vi "Begin.vi"(8 "error in":errorcluster) -> (0 "error out":errorcluster)   [LabVIEW 2017]
doc: "Called before other user functions, this VI is expected to open initial I/O refnums, load in file data, and do all program initialization. Notice that the <B>error out</B> terminal is simply used for data flow. Wiring it to other structures or subVIs ensures that this VI runs first."
uses:
  <vilib>/Rock Robotics/WPI/DriverStation/WPI_DriverStationRobotMode2.ctl
  <vilib>/Rock Robotics/WPI/Joystick/WPI_JoystickDeviceEnum.ctl
  <vilib>/Rock Robotics/WPI/Solenoid/WPI_SolenoidChannel.ctl
  <vilib>/Rock Robotics/WPI/SafetyOutput/WPI_SafetyOutputConfigMenu.ctl
  <vilib>/Rock Robotics/SystemInterfaces/DIO/FPGA_DIOPWMChannel.ctl
  Robot Global Data.vi
  <vilib>/Rock Robotics/Network Tables/NT Write String Array.vi
  <vilib>/Rock Robotics/WPI/MotorControl/WPI_MotorControlOpen VictorSP.vi
  <vilib>/Rock Robotics/WPI/Solenoid/WPI_SolenoidOpenDouble.vi
  <vilib>/Rock Robotics/WPI/RobotDrive/WPI_RobotDriveOpen2MotorWithExistingMotors.vi
  <vilib>/Rock Robotics/WPI/Utilities/WPI_GetSetVariantRefNum.vi
  <vilib>/Rock Robotics/WPI/MotorControl/WPI_MotorControlOpen SPARK.vi
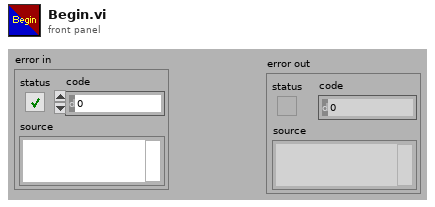
[diagram p1: front panel]
types:
  T1 = typedef "FPGA_DIOPWMChannel.ctl" = enum8{"PWM 0", "PWM 1", "PWM 2", "PWM 3", "PWM 4", "PWM 5", "PWM 6", "PWM 7", "PWM 8", "PWM 9", "PWM MXP 0", "PWM MXP 1", "PWM MXP 2", "PWM MXP 3", "PWM MXP 4", "PWM MXP 5", "PWM MXP 6", "PWM MXP 7", "PWM MXP 8", "PWM MXP 9", "Invalid"}
  T2 = typedef "WPI_SafetyOutputConfigMenu.ctl" = enum16{"Enable", "Disable"}
  T3 = typedef "WPI_SolenoidChannel.ctl" = enum8{"Solenoid 0", "Solenoid 1", "Solenoid 2", "Solenoid 3", "Solenoid 4", "Solenoid 5", "Solenoid 6", "Solenoid 7", "Invalid"}
  T4 = typedef "WPI_JoystickDeviceEnum.ctl" = enum16{"USB 0", "USB 1", "USB 2", "USB 3", "USB 4", "USB 5"}
  T5 = typedef "WPI_DriverStationRobotMode2.ctl" = enum16{"Autonomous Disabled", "Autonomous Enabled", "Teleop Disabled", "Teleop Enabled", "Disconnected", "Finish", "Test Disabled", "Test Enabled", "Emergency Stopped"}
  T6 = typedef "WPI_MotorControlDeviceRef.ctl" = cluster{"DeviceStatus":errorcluster, "Type":T7, "PWM":cluster{"PWM Channel":T1, "DeadBand":T8}, "CAN":cluster{"Device Number":u8, "SetOutput VI Ref":variant, "GetOutput VI Ref":variant, "Enable VI Ref":variant, "Disable VI Ref":variant, "Data":variant}, "Invert":bool, "DIO PWM":cluster{"PWM \"Enable\" Channel":T1, "DIOChannel":T9, "PWM Rate":dbl}}
  T7 = typedef "WPI_MotorControlType.ctl" = enum16{"PWM", "CAN", "DIO PWM"}
  T8 = typedef "WPI_PWMDeadband.ctl" = cluster{"Name":string, "maxPositivePwm":i32, "minPositivePwm":i32, "centerPwm":i32, "maxNegativePwm":i32, "minNegativePwm":i32, "angularRange":u16}
  T9 = typedef "FPGA_DIOChannel.ctl" = enum8{"DIO 0", "DIO 1", "DIO 2", "DIO 3", "DIO 4", "DIO 5", "DIO 6", "DIO 7", "DIO 8", "DIO 9", "DIO MXP 0", "DIO MXP 1", "DIO MXP 2", "DIO MXP 3", "DIO MXP 4", "DIO MXP 5", "DIO MXP 6", "DIO MXP 7", "DIO MXP 8", "DIO MXP 9", "DIO MXP 10", "DIO MXP 11", "DIO MXP 12", "DIO MXP 13", "DIO MXP 14", "DIO MXP 15", "SPI Port CS1", "SPI Port CS2", "SPI Port CS3", "SPI Port MISO", "SPI Port MOSI", "Invalid"}
  T10 = typedef "WPI_SolenoidDevRef.ctl" = cluster{"DevStatus":errorcluster, "Pneumatics Control Module":u8, "Forward Solenoid Channel":T3, "Reverse Solenoid Channel":T3}
  T11 = typedef "WPI_JoystickDevRef.ctl" = cluster{"Device":T4}
  T12 = typedef "WPI_RobotDriveDevRef.ctl" = cluster{"DevStatus":errorcluster, "Motors[]":T6[], "Square Inputs":bool, "Max Output":dbl}
  T13 = typedef "WPI_CompressorDevRef.ctl" = cluster{"DevStatus":errorcluster, "Pneumatics Control Module":u8}
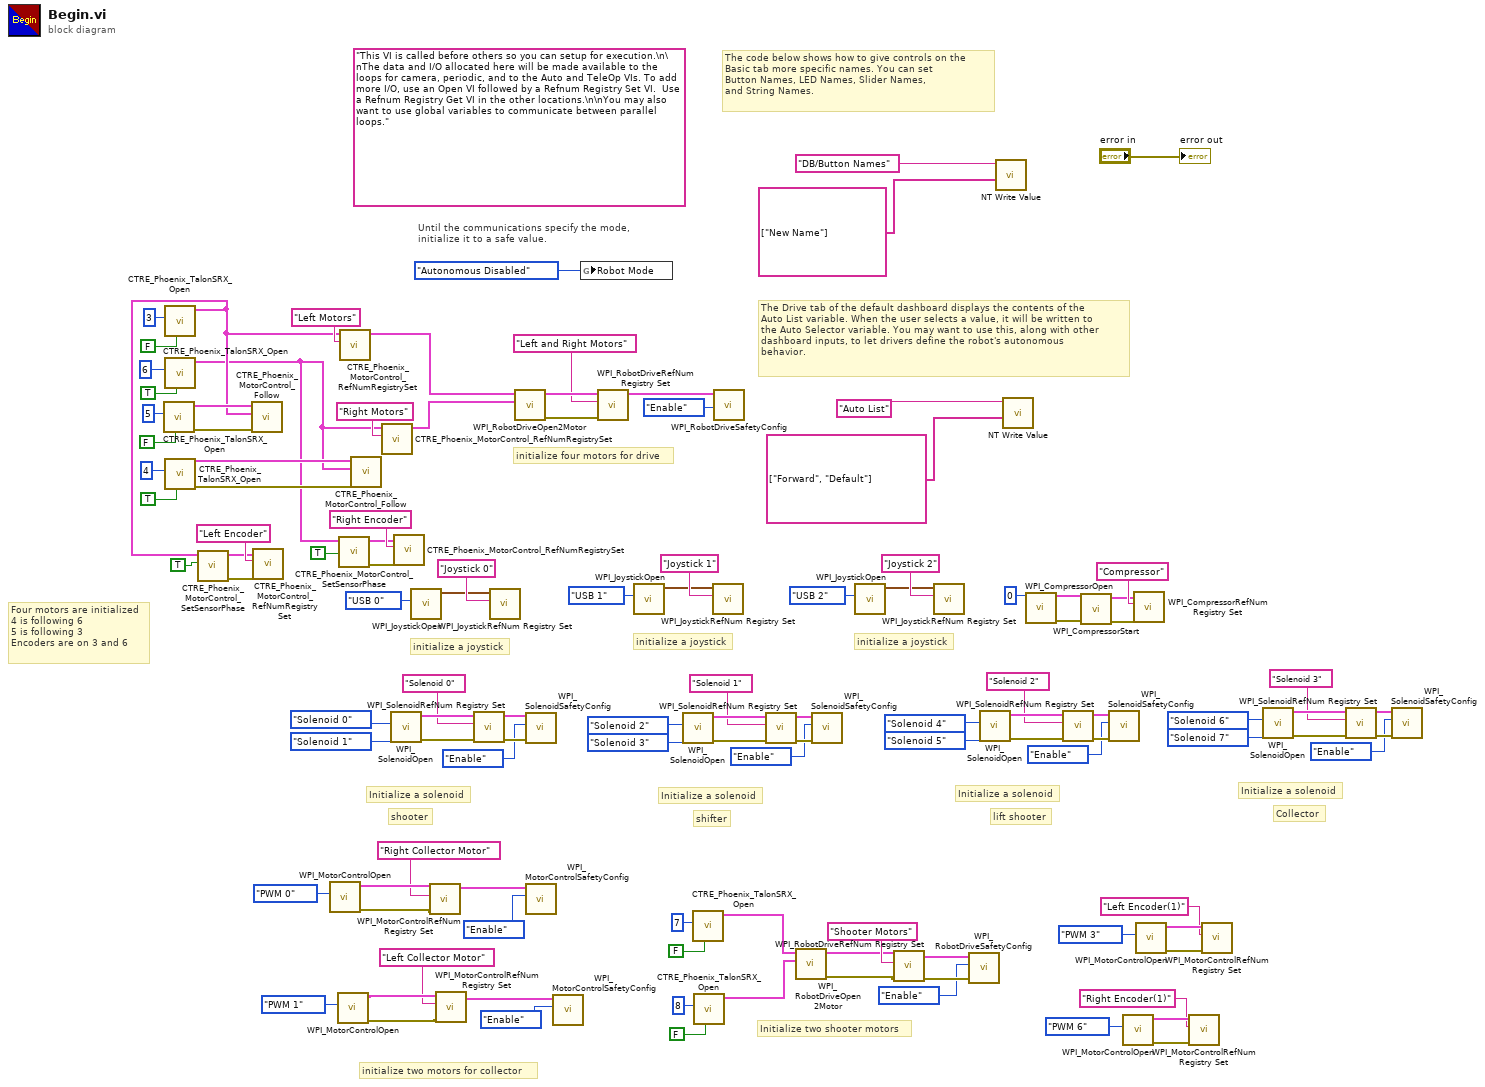
[diagram p0: block diagram]
diagram:
  (unwired) "This VI is called before others so you can setup for execution.\n\nThe data and I/O allocated here will be made available to the loops for camera, periodic, and to the Auto and TeleOp VIs. To add more I/O, use an Open VI followed by a Refnum Registry Set VI.  Use a Refnum Registry Get VI in the other locations.\n\nYou may also want to use global variables to communicate between parallel loops."
  # "Four motors are initialized\n4 is following 6\n5 is following 3\nEncoders are on 3 and 6"
  # "Initialize two shooter motors"
  # "Collector"
  # "Initialize a solenoid"
  # "lift shooter"
  # "Initialize a solenoid"
  # "initialize two motors for collector"
  # "shifter"
  # "shooter"
  # "Initialize a solenoid"
  # "Initialize a solenoid"
  # "initialize a joystick"
  # "initialize a joystick"
  # "The Drive tab of the default dashboard displays the contents of the\nAuto List variable. When the user selects a value, it will be written to\nthe Auto Selector variable. You may want to use this, along with other\ndashboard inputs, to let drivers define the robot's autonomous\nbehavior."
  # "The code below shows how to give controls on the\nBasic tab more specific names. You can set\nButton Names, LED Names, Slider Names,\nand String Names."
  # "initialize a joystick"
  # "Until the communications specify the mode,\ninitialize it to a safe value."
  # "initialize four motors for drive"
  n1 = call <vilib>:"CTRE_Phoenix_TalonSRX_Open.vi"("Invert"=FALSE, "Device Number"=u8 5) -> ("error out"=w56:errorcluster, "CAN Talon SRX Ref"=w55:T6)  [unwired: 8 in]
  n2 = call <vilib>:"CTRE_Phoenix_TalonSRX_Open.vi"("Invert"=FALSE, "Device Number"=u8 3) -> ("CAN Talon SRX Ref"=w43:T6)  [unwired: 8 in, 1 out]
  n3 = call <vilib>:"CTRE_Phoenix_TalonSRX_Open.vi"("Invert"=TRUE, "Device Number"=u8 6) -> ("CAN Talon SRX Ref"=w39:T6)  [unwired: 8 in, 1 out]
  n4 = call <vilib>:"CTRE_Phoenix_TalonSRX_Open.vi"("Invert"=TRUE, "Device Number"=u8 4) -> ("error out"=w53:errorcluster, "CAN Talon SRX Ref"=w54:T6)  [unwired: 8 in]
  n5 = call <vilib>:"CTRE_Phoenix_MotorControl_SetSensorPhase.vi"("PhaseSensor"=TRUE ("Invert"), "PhoenixMotorControlDevRef"=w43) -> ("error out"=w44:errorcluster, "PhoenixMotorControlDevRef"=w45:T6)  [unwired: 8 in]
  n6 = call <vilib>:"CTRE_Phoenix_MotorControl_Follow.vi"("error in (no error)"=w56, "Master Controller to Follow"=w43, "PhoenixMotorControlDevRef"=w55) -> ()  [unwired: 7 in, 2 out]
  n7 = call "CTRE_Phoenix_MotorControl_RefNumRegistrySet.vi"("error in (no error)"=w44, "refnum name"="Left Encoder", "PhoenixMotorControlDevRef"=w45) -> ()  [unwired: 7 in, 2 out]
  n8 = call-poly <vilib>:"WPI_MotorControlOpen.vi"("PWM Channel"=FPGA_DIOPWMChannel."PWM 0") -> ("error out"=w68:errorcluster, "MotorControlDeviceRef"=w72:T6)  [unwired: 9 in]
  n9 = call-poly <vilib>:"WPI_MotorControlOpen.vi"("PWM Channel"=FPGA_DIOPWMChannel."PWM 1") -> ("error out"=w63:errorcluster, "MotorControlDeviceRef"=w67:T6)  [unwired: 9 in]
  n10 = call <vilib>:"CTRE_Phoenix_MotorControl_SetSensorPhase.vi"("PhaseSensor"=TRUE ("Invert"), "PhoenixMotorControlDevRef"=w39) -> ("error out"=w40:errorcluster, "PhoenixMotorControlDevRef"=w41:T6)  [unwired: 8 in]
  n11 = call "CTRE_Phoenix_MotorControl_RefNumRegistrySet.vi"("refnum name"="Left Motors", "PhoenixMotorControlDevRef"=w43) -> ("PhoenixMotorControlDevRef"=w60:T6)  [unwired: 8 in, 1 out]
  n12 = call <vilib>:"CTRE_Phoenix_MotorControl_Follow.vi"("error in (no error)"=w53, "Master Controller to Follow"=w39, "PhoenixMotorControlDevRef"=w54) -> ()  [unwired: 7 in, 2 out]
  n13 = call "CTRE_Phoenix_MotorControl_RefNumRegistrySet.vi"("refnum name"="Right Motors", "PhoenixMotorControlDevRef"=w39) -> ("PhoenixMotorControlDevRef"=w59:T6)  [unwired: 8 in, 1 out]
  n14 = call-poly <vilib>:"WPI_SolenoidOpen.vi"("Reverse Solenoid Channel"=WPI_SolenoidChannel."Solenoid 1", "Forward Solenoid Channel"=WPI_SolenoidChannel."Solenoid 0" ("Solenoid Channel")) -> ("error out"=w87:errorcluster, "SolenoidDevRef"=w86:T10)  [unwired: 8 in]
  n15 = call "CTRE_Phoenix_MotorControl_RefNumRegistrySet.vi"("error in (no error)"=w40, "refnum name"="Right Encoder", "PhoenixMotorControlDevRef"=w41) -> ()  [unwired: 7 in, 2 out]
  n16 = call <vilib>:"WPI_JoystickOpen.vi"("JoystickDevice"=WPI_JoystickDeviceEnum."USB 0") -> ("JoystickDevRef"=w109:T11)  [unwired: 10 in]
  n17 = call <vilib>:"WPI_MotorControlRefNum Registry Set.vi"("error in (no error)"=w68, "refnum name"="Right Collector Motor", "MotorControlDevRef"=w72) -> ("MotorControlDevRef"=w70:T6)  [unwired: 7 in, 1 out]
  n18 = call <vilib>:"WPI_MotorControlRefNum Registry Set.vi"("error in (no error)"=w63, "refnum name"="Left Collector Motor", "MotorControlDevRef"=w67) -> ("MotorControlDevRef"=w65:T6)  [unwired: 7 in, 1 out]
  n19 = call <vilib>:"WPI_SolenoidRefNum Registry Set.vi"("error in (no error)"=w87, "refnum name"="Solenoid 0", "SolenoidDevRef"=w86) -> ("error out"=w80:errorcluster, "SolenoidDevRef"=w79:T10)  [unwired: 7 in]
  n20 = call <vilib>:"WPI_JoystickRefNum Registry Set.vi"("refnum name"="Joystick 0", "JoystickDevRef"=w109) -> ()  [unwired: 8 in, 2 out]
  n21 = call-poly <vilib>:"WPI_RobotDriveOpen2Motor.vi"("Right Motor Dev Ref"=w59, "Left Motor Dev Ref"=w60) -> ("error out"=w114:errorcluster, "RobotDriveDevRef"=w116:T12)  [unwired: 8 in]
  n22 = call <vilib>:"WPI_SolenoidSafetyConfig.vi"("error in (no error)"=w80, "mode"=WPI_SafetyOutputConfigMenu."Enable", "SolenoidDevRef"=w79) -> ()  [unwired: 7 in, 2 out]
  n23 = call <vilib>:"WPI_MotorControlSafetyConfig.vi"("mode"=WPI_SafetyOutputConfigMenu."Enable", "MotorControlDevRef"=w70) -> ()  [unwired: 8 in, 2 out]
  n24 = call <vilib>:"WPI_MotorControlSafetyConfig.vi"("mode"=WPI_SafetyOutputConfigMenu."Enable", "MotorControlDevRef"=w65) -> ()  [unwired: 8 in, 2 out]
  n25 = global write "Robot Global Data.vi" "Robot Mode"(WPI_DriverStationRobotMode2."Autonomous Disabled" ("Robot Mode")) -> ()
  n26 = call <vilib>:"WPI_RobotDriveRefNum Registry Set.vi"("error in (no error)"=w114, "refnum name"="Left and Right Motors", "RobotDriveDevRef"=w116) -> ("RobotDriveDevRef"=w113:T12)  [unwired: 1 in, 7 out]
  n27 = call <vilib>:"WPI_JoystickOpen.vi"("JoystickDevice"=WPI_JoystickDeviceEnum."USB 1") -> ("JoystickDevRef"=w94:T11)  [unwired: 10 in]
  n28 = call-poly <vilib>:"WPI_SolenoidOpen.vi"("Reverse Solenoid Channel"=WPI_SolenoidChannel."Solenoid 3", "Forward Solenoid Channel"=WPI_SolenoidChannel."Solenoid 2" ("Solenoid Channel")) -> ("error out"=w83:errorcluster, "SolenoidDevRef"=w82:T10)  [unwired: 8 in]
  n29 = call <vilib>:"CTRE_Phoenix_TalonSRX_Open.vi"("Invert"=FALSE, "Device Number"=u8 7) -> ("CAN Talon SRX Ref"=w10:T6)  [unwired: 8 in, 1 out]
  n30 = call <vilib>:"CTRE_Phoenix_TalonSRX_Open.vi"("Invert"=FALSE, "Device Number"=u8 8) -> ("CAN Talon SRX Ref"=w9:T6)  [unwired: 8 in, 1 out]
  n31 = call <vilib>:"WPI_JoystickRefNum Registry Set.vi"("refnum name"="Joystick 1", "JoystickDevRef"=w94) -> ()  [unwired: 8 in, 2 out]
  n32 = call <vilib>:"WPI_RobotDriveSafetyConfig.vi"("mode"=WPI_SafetyOutputConfigMenu."Enable", "RobotDriveDevRef"=w113) -> ()  [unwired: 8 in, 2 out]
  n33 = call <vilib>:"WPI_SolenoidRefNum Registry Set.vi"("error in (no error)"=w83, "refnum name"="Solenoid 1", "SolenoidDevRef"=w82) -> ("error out"=w77:errorcluster, "SolenoidDevRef"=w76:T10)  [unwired: 7 in]
  n34 = call-poly <vilib>:"WPI_RobotDriveOpen2Motor.vi"("Right Motor Dev Ref"=w9, "Left Motor Dev Ref"=w10) -> ("error out"=w11:errorcluster, "RobotDriveDevRef"=w12:T12)  [unwired: 8 in]
  n35 = call <vilib>:"WPI_SolenoidSafetyConfig.vi"("error in (no error)"=w77, "mode"=WPI_SafetyOutputConfigMenu."Enable", "SolenoidDevRef"=w76) -> ()  [unwired: 7 in, 2 out]
  n36 = call <vilib>:"WPI_JoystickOpen.vi"("JoystickDevice"=WPI_JoystickDeviceEnum."USB 2") -> ("JoystickDevRef"=w97:T11)  [unwired: 10 in]
  n37 = call <vilib>:"WPI_RobotDriveRefNum Registry Set.vi"("error in (no error)"=w11, "refnum name"="Shooter Motors", "RobotDriveDevRef"=w12) -> ("error out"=w14:errorcluster, "RobotDriveDevRef"=w15:T12)  [unwired: 7 in]
  n38 = call <vilib>:"WPI_JoystickRefNum Registry Set.vi"("refnum name"="Joystick 2", "JoystickDevRef"=w97) -> ()  [unwired: 8 in, 2 out]
  n39 = call <vilib>:"WPI_RobotDriveSafetyConfig.vi"("error in (no error)"=w14, "mode"=WPI_SafetyOutputConfigMenu."Enable", "RobotDriveDevRef"=w15) -> ()  [unwired: 7 in, 2 out]
  n40 = call-poly <vilib>:"WPI_SolenoidOpen.vi"("Reverse Solenoid Channel"=WPI_SolenoidChannel."Solenoid 5", "Forward Solenoid Channel"=WPI_SolenoidChannel."Solenoid 4" ("Solenoid Channel")) -> ("error out"=w35:errorcluster, "SolenoidDevRef"=w34:T10)  [unwired: 8 in]
  n41 = call-poly <vilib>:"NT Write Value.vi"("String Array"=string[] ["New Name"], "Name"="DB/Button Names") -> ()  [unwired: 9 in, 1 out]
  n42 = call-poly <vilib>:"NT Write Value.vi"("String Array"=string[] ["Forward", "Default"], "Name"="Auto List") -> ()  [unwired: 9 in, 1 out]
  n43 = call <vilib>:"WPI_CompressorOpen.vi"("Pneumatics Control Module (0)"=u8 0) -> ("CompressorDevRef"=w51:T13, "error out"=w50:errorcluster)  [unwired: 13 in]
  n44 = call <vilib>:"WPI_SolenoidRefNum Registry Set.vi"("error in (no error)"=w35, "refnum name"="Solenoid 2", "SolenoidDevRef"=w34) -> ("error out"=w32:errorcluster, "SolenoidDevRef"=w31:T10)  [unwired: 7 in]
  n45 = call <vilib>:"WPI_CompressorStart.vi"("error in (no error)"=w50, "CompressorDevRef"=w51) -> ("error out"=w47:errorcluster, "CompressorDevRef"=w48:T13)  [unwired: 8 in]
  n46 = call <vilib>:"WPI_SolenoidSafetyConfig.vi"("error in (no error)"=w32, "mode"=WPI_SafetyOutputConfigMenu."Enable", "SolenoidDevRef"=w31) -> ()  [unwired: 7 in, 2 out]
  n47 = call-poly <vilib>:"WPI_MotorControlOpen.vi"("PWM Channel"=FPGA_DIOPWMChannel."PWM 6") -> ("error out"=w3:errorcluster, "MotorControlDeviceRef"=w2:T6)  [unwired: 9 in]
  n48 = call <vilib>:"WPI_CompressorRefNum Registry Set.vi"("error in (no error)"=w47, "refnum name"="Compressor", "CompressorDevRef"=w48) -> ()  [unwired: 7 in, 2 out]
  n49 = call-poly <vilib>:"WPI_MotorControlOpen.vi"("PWM Channel"=FPGA_DIOPWMChannel."PWM 3") -> ("error out"=w7:errorcluster, "MotorControlDeviceRef"=w6:T6)  [unwired: 9 in]
  n50 = call <vilib>:"WPI_MotorControlRefNum Registry Set.vi"("error in (no error)"=w3, "refnum name"="Right Encoder(1)", "MotorControlDevRef"=w2) -> ()  [unwired: 7 in, 2 out]
  n51 = call <vilib>:"WPI_MotorControlRefNum Registry Set.vi"("error in (no error)"=w7, "refnum name"="Left Encoder(1)", "MotorControlDevRef"=w6) -> ()  [unwired: 7 in, 2 out]
  n52 = call-poly <vilib>:"WPI_SolenoidOpen.vi"("Reverse Solenoid Channel"=WPI_SolenoidChannel."Solenoid 7", "Forward Solenoid Channel"=WPI_SolenoidChannel."Solenoid 6" ("Solenoid Channel")) -> ("error out"=w27:errorcluster, "SolenoidDevRef"=w26:T10)  [unwired: 8 in]
  n53 = call <vilib>:"WPI_SolenoidRefNum Registry Set.vi"("error in (no error)"=w27, "refnum name"="Solenoid 3", "SolenoidDevRef"=w26) -> ("error out"=w24:errorcluster, "SolenoidDevRef"=w23:T10)  [unwired: 7 in]
  n54 = call <vilib>:"WPI_SolenoidSafetyConfig.vi"("error in (no error)"=w24, "mode"=WPI_SafetyOutputConfigMenu."Enable", "SolenoidDevRef"=w23) -> ()  [unwired: 7 in, 2 out]
  "error out" <- "error in"
